vi "Replace IO Controls.vi"(0 "VI in":refnum<vi>, 11 "error in (no error)":errorcluster) -> (4 "VI out":refnum<vi>, 15 "error out":errorcluster)   [LabVIEW 2021, in "Migrator.lvlib"]
uses:
  Migrator.lvlib
  <vilib>/Utility/traverseref.llb/TRef TravTarget.ctl
  <vilib>/Utility/traverseref.llb/VI Scripting - Traverse.lvlib
  Migrator Reusables/Migrator Reusables.lvlib
  Path Functions/Path Functions.lvlib
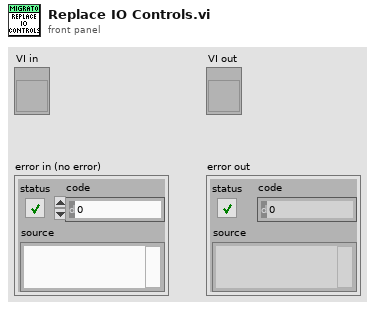
[diagram p1: front panel]
types:
  T1 = typedef "TRef TravTarget.ctl" = enum16{"FP", "BD", "Other"}
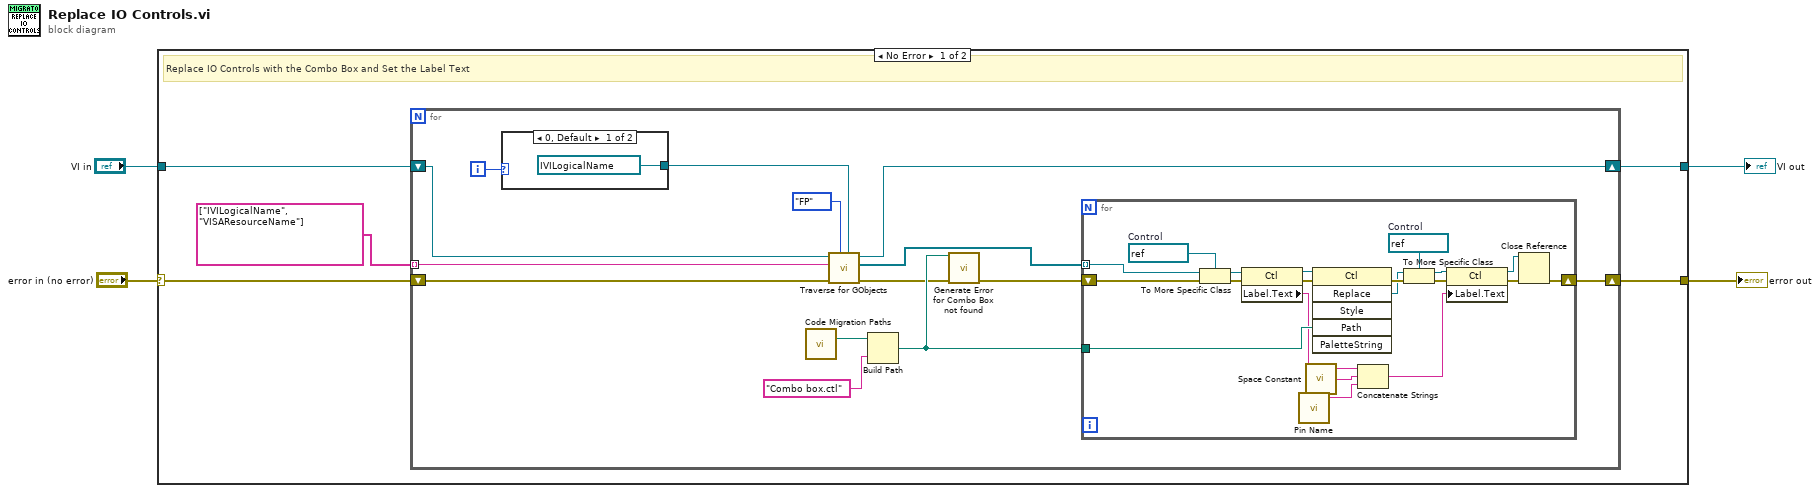
[diagram p0: block diagram]
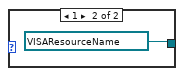
[diagram p2: hidden frame]
diagram:
  n1 = case shown="No Error" "error in (no error)" {
    selector: "error in (no error)" -> [w7 w46]
    tunnel: [w5 w46] -> w4
    tunnel: [w9 w47] -> w3
    tunnel: "VI in" -> [w6 w47]
    frame No Error {
      # "Replace IO Controls with the Combo Box and Set the Label Text"
      n2 = for {
        tunnel: string[] ["IVILogicalName", "VISAResourceName"] ("Class Name") -> [w21] mode=indexing
        shift-right: [w12] -> w5
        shift-left: w7 -> [w20]
        shift-right: [w22] -> w9
        shift-left: w6 -> [w19]
        i -> [w11]
        n3 = case shown="0, Default" w11 {
          tunnel: [refnum<vi> refnum ("Other Refnum") refnum<vi> refnum ("Other Refnum")] -> w10
          frame 0, Default {
          }
          frame 1 {
          }
        }
        n4 = call "Code Migration Paths.vi"() -> ("IO Controls"=w18:path)  [unwired: 7 in, 8 out]
        n5 = call <vilib>:"Traverse for GObjects.vi"("Other Refnum"=w10, "Traverse Target"=TRef_TravTarget."FP", "error in (no error)"=w20, "Class Name"=w21, "VI Refnum"=w19) -> ("error out"=w15:errorcluster, "References"=w13:refnum<vi>[], "dup VI Refnum"=w22:refnum<vi>)  [unwired: 3 in, 1 out]
        n6 = Build Path(base path=w18, name or relative path="Combo box.ctl" ("string")) -> (appended path=w16:path)
        n7 = call "Generate Error for Combo Box not found.vi"("Template combox path"=w16, "error in (no error)"=w15) -> ("error out"=w14:errorcluster)  [unwired: 13 in]
        n8 = for {
          tunnel: w13 -> [w44] mode=indexing
          tunnel: w16 -> [w45]
          shift-right: [w26] -> w12
          shift-left: w14 -> [w43]
          w37 = refnum<vi> refnum  # Control
          w42 = refnum<vi> refnum  # Control
          n9 = To More Specific Class(target class=w42, reference=w44, error in=w43) -> (specific class reference=w41:refnum<vi>, error out=w39:errorcluster)
          n10 = property class="Ctl"(reference=w41, error in=w39) -> (reference out=w40:refnum<vi>, error out=w38:errorcluster, "Label.Text"=w30:string)
          n11 = call "Pin Name.vi"() -> ("Pin Name"=w31:string)  [unwired: 5 in]
          n12 = call <vilib>:"Space Constant.vi"() -> ("String"=w32:string)
          n13 = invoke class="Ctl" method="Replace"(reference=w40, error in=w38, "Path"=w45) -> (error out=w36:errorcluster, "Replace"=w35:refnum<vi>)  [unwired: 3 in, 4 out]
          n14 = Concatenate Strings(w30, w32, w31) -> (w29:string)
          n15 = To More Specific Class(target class=w37, reference=w35, error in=w36) -> (specific class reference=w34:refnum<vi>, error out=w33:errorcluster)
          n16 = property class="Ctl"(reference=w34, error in=w33, "Label.Text"=w29) -> (reference out=w27:refnum<vi>, error out=w28:errorcluster)
          n17 = Close Reference(reference=w27, error in (no error)=w28) -> (error out=w26:errorcluster)
        }
      }
    }
    frame Error {
    }
  }
  "error out" <- w4
  "VI out" <- w3
